vi "History Get All.vi"(6 "Descending? (F)":bool, 8 "error in (no error)":errorcluster, 10 "Sort by (sVersion)":T1=enum."sVersion", 11 "Connection Refnum":T2) -> (0 "error out":errorcluster, 1 "Versions":string[](array[string]), 2 "History Records":T3[](array[typedef]), 3 "Connection Refnum":T2, 4 "Data Present":bool)   [LabVIEW 2011]
uses:
  History Record.ctl
  Summitek EXT/ODBC/SQL Controls/Connection Refnum.ctl
  History Fields.ctl
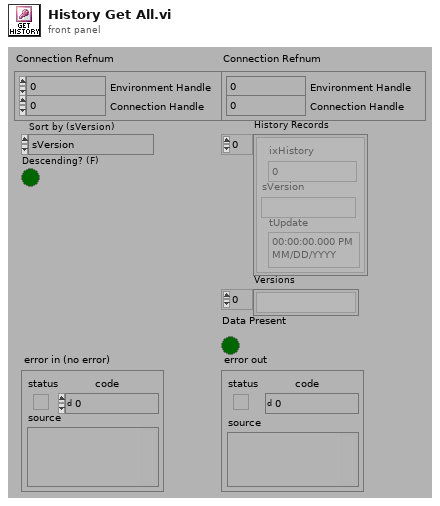
[diagram p1: front panel]
types:
  T1 = typedef "History Fields.ctl" = enum32{"ixHistory", "sVersion", "tUpdate"}
  T2 = typedef "Connection Refnum.ctl" = cluster{"Environment Handle":i32, "Connection Handle":i32}
  T3 = typedef "History Record.ctl" = cluster{"ixHistory":i32, "sVersion":string, "tUpdate":timestamp}
  T4 = typedef "Statement Refnum.ctl" = cluster{"Statement Handle":i32, "Parameter Number":u16}
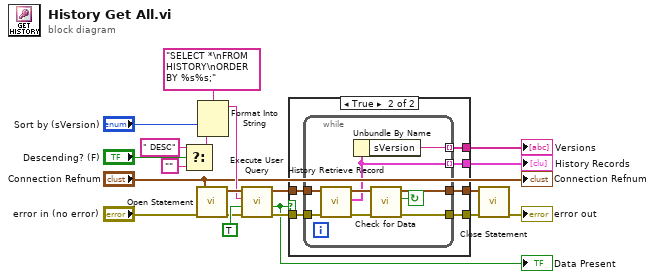
[diagram p0: block diagram]
diagram:
  n1 = Select(t=" DESC" ("input 2"), s="Descending? (F)", f="") -> (s? t:f=w10:string)
  n2 = call "Open Statement.vi"("error in (no error)"="error in (no error)", "Connection Refnum"="Connection Refnum") -> ("error out"=w14:errorcluster, "Statement Refnum"=w15:T4)  [unwired: 4 out]
  n3 = Format Into String(format string="SELECT *\nFROM HISTORY\nORDER BY %s%s;" ("Query Name"), "Sort by (sVersion)", w10) -> (resulting string=w6:string)  [unwired: 2 in, 1 out]
  n4 = call "Execute User Query.vi"("error in (no error)"=w14, "Return Data? (f)"=TRUE, "User Query"=w6, "Statement Refnum"=w15) -> ("error out"=w20:errorcluster, "Data Present?"=w13:bool, "Statement Refnum"=w19:T4)  [unwired: 1 out]
  "Data Present" <- w13
  n5 = case shown="True" w13 {
    tunnel: w20 -> [w21 w27]
    tunnel: w19 -> [w22 w28]
    tunnel: [w21 w25] -> w16
    tunnel: [w22 w26] -> w17
    tunnel: [_ w24] -> w3
    tunnel: [_ w23] -> w2
    frame False {
    }
    frame True {
      n6 = while {
        tunnel: w28 -> [w36]
        tunnel: w27 -> [w35]
        tunnel: [w33] -> w26
        tunnel: [w31] -> w25
        tunnel: [w30] -> w23 mode=indexing
        tunnel: [w29] -> w24 mode=indexing
        stop <- w37 continue-if-true
        n7 = call "History Retrieve Record.vi"("error in (no error)"=w35, "Statement Refnum"=w36) -> ("error out"=w32:errorcluster, "History Record"=w30:T3, "Statement Refnum"=w34:T4)  [unwired: 7 out]
        n8 = Unbundle By Name(w30) -> ("sVersion"=w29:string)
        n9 = call "Check for Data.vi"("error in (no error)"=w32, "Statement Refnum"=w34) -> ("error out"=w31:errorcluster, "Data Present?"=w37:bool, "Statement Refnum"=w33:T4)  [unwired: 3 out]
      }
    }
  }
  "History Records" <- w2
  "Versions" <- w3
  n10 = call "Close Statement.vi"("error in (no error)"=w16, "Statement Refnum"=w17) -> ("error out"=→"error out":errorcluster)  [unwired: 5 out]
  "Connection Refnum" <- "Connection Refnum"
